vi "读取历史数据.vi"(0 "file path (dialog if empty)":path caption="文件路径 （空时为对话框）", 11 "error in (no error)":errorcluster caption="错误输入（无错误）") -> (4 "Title":string[](array[string]), 6 "Data":string[][](array[string]), 8 "行首字符串":string[](array[string]), 10 "数据波形图":dbl[][](graph), 15 "error out":errorcluster caption="错误输出")   [LabVIEW 2017]
uses:
  <vilib>/Utility/file.llb/Read Delimited Spreadsheet (string).vi
panel:
  out "添加的数组":dbl[][](array[numeric])
  out "大小":i32[](array[numeric])
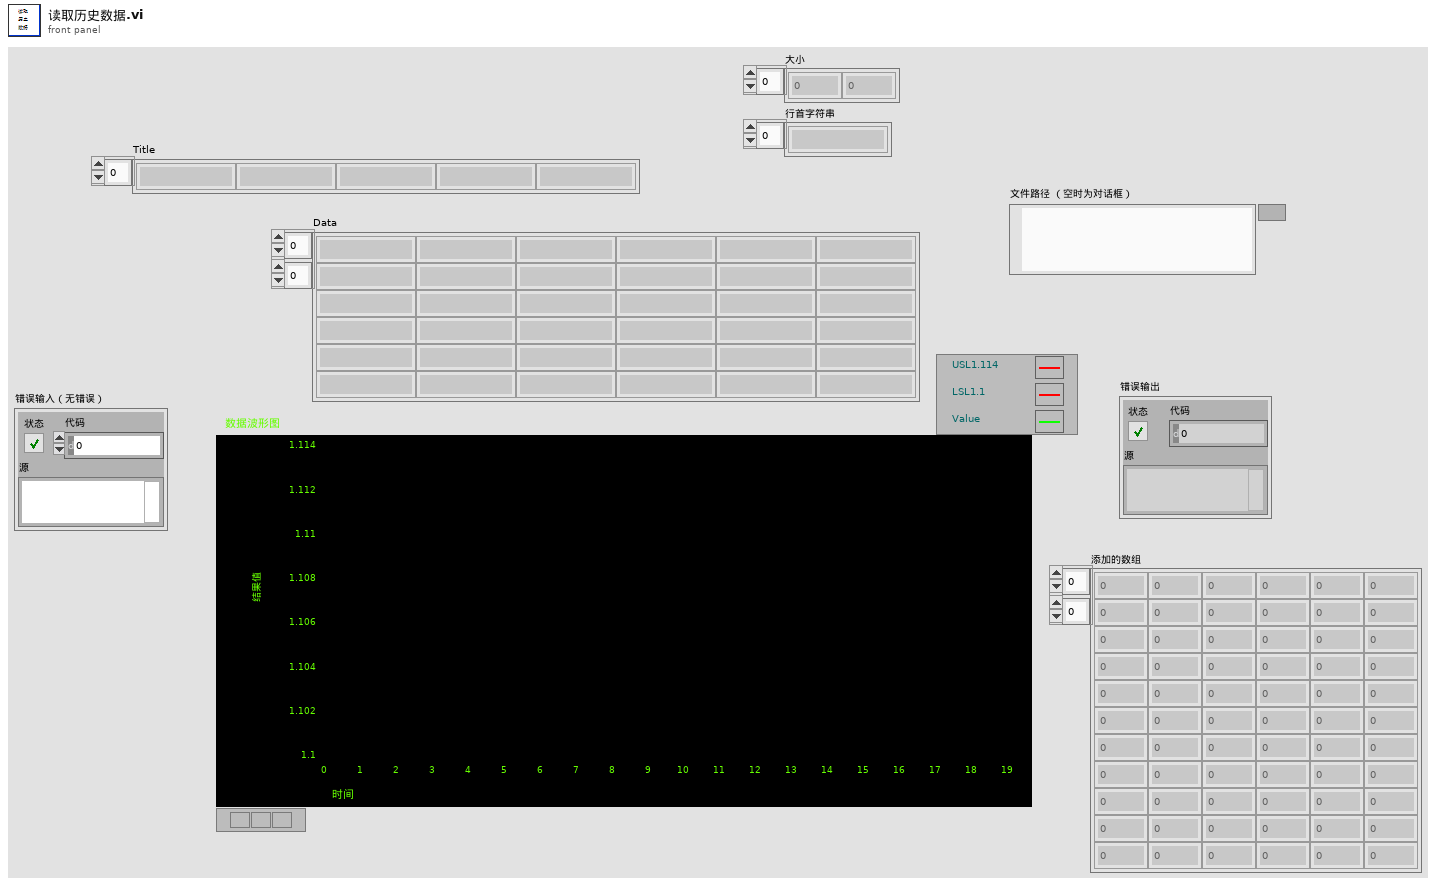
[diagram p1: front panel]
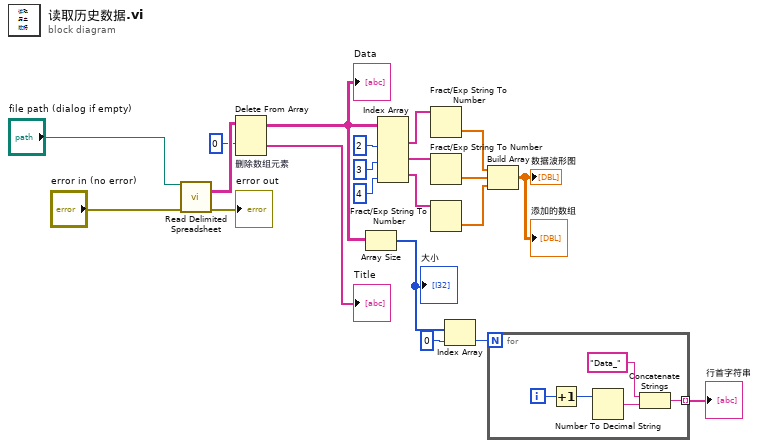
[diagram p0: block diagram]
diagram:
  n1 = call-poly <vilib>:"Read Delimited Spreadsheet.vi"("file path (dialog if empty)"="file path (dialog if empty)", "error in (no error)"="error in (no error)") -> ("all rows"=w20:string[][], "error out"=→"error out":errorcluster)  [unwired: 8 in, 4 out]
  n2 = Delete From Array "删除数组元素"(array=w20, index (row)=0 ("索引 (行)")) -> (deleted portion=→"Title":string[], array with subset deleted=w11:string[][])  [unwired: 2 in]
  "Data" <- w11
  n3 = Array Size(array=w11) -> (size(s)=w15:i32[])
  "大小" <- w15
  n4 = Index Array(array=w11, index (col) #1=2 ("禁用的索引 (列)"), index (col) #2=3 ("索引 (列)"), index (col) #3=4 ("索引 (列)")) -> (element #1=w7:string[], element #2=w6:string[], element #3=w5:string[])  [unwired: 3 in]
  n5 = Fract/Exp String To Number(string=w7) -> (number=w4:dbl[])  [unwired: 3 in, 1 out]
  n6 = Fract/Exp String To Number(string=w6) -> (number=w3:dbl[])  [unwired: 3 in, 1 out]
  n7 = Fract/Exp String To Number(string=w5) -> (number=w2:dbl[])  [unwired: 3 in, 1 out]
  n8 = Index Array(array=w15, index=0 ("索引")) -> (element=w13:i32)
  n9 = Build Array(w4, w3, w2) -> (→"数据波形图" →"添加的数组":dbl[][])
  n10 = for {
    N: w13 -> [_]
    tunnel: [w22] -> w12 mode=indexing
    i -> [w26]
    n11 = Increment(x=w26) -> (x+1=w25:i32)
    n12 = Number To Decimal String(number=w25) -> (decimal integer string=w23:string)  [unwired: 1 in]
    n13 = Concatenate Strings("Data_" ("字符串"), w23) -> (w22:string)
  }
  "行首字符串" <- w12
